vi "Process.vi"(8 "error in":errorcluster, 11 "XYStage":refnum<class "XYStage.lvclass">) -> (0 "error out":errorcluster, 3 "XYStage out":refnum<class "XYStage.lvclass">)   [LabVIEW 2020, in "XYStage.lvclass"]
doc: "---------------------------------------------------------------\nJKI State Machine Objects™\nhttp://jki.net/state-machine-objects/\nCopyright (C) 2005-2015, JKI <info@jki.net>\nALL RIGHTS RESERVEDJKI State Machine Objects (SMO) 1.0.0.5\nJKI - JKI\nCopyright (c) 2016, JKI"
uses:
  XYStage.lvclass
  XYStage.lvclass/XYStage.ctl
  <vilib>/JKI/JKI SMO/SMO/SMO.lvclass
  <vilib>/JKI/JKI SMO/SMO/Typedefs/Parent Call--Enum.ctl
  Typedefs/(real)Coords--Cluster.ctl
  C:/Program Files/National Instruments/LabVIEW 2020/vi.lib/JKI/JKI SMO/SMO/SMO.lvclass
  C:/Users/huipeng8/Desktop/SMO-HAL-Webinar/Subsystems/XYStage/XYStage.lvclass
panel:
  # "For instructions on how to use the JKI State Machine Objects, examples and video tutorials, visit:\nhttp://jki.net/state-machine-objects/\n\nJKI State Machine Objects™\nhttp://jki.net/state-machine-objects/\nCopyright (C) 2005-2015, JKI <info@jki.net>\nALL RIGHTS RESERVED"
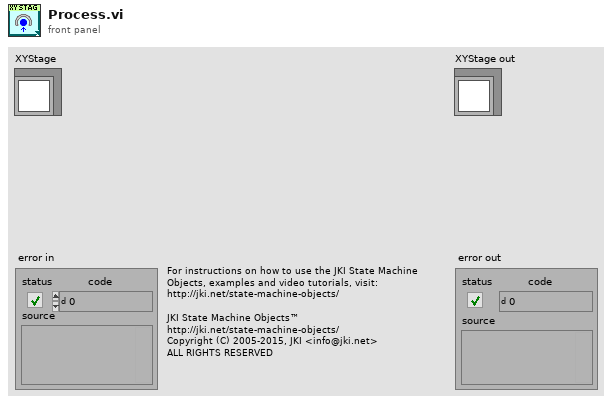
[diagram p1: front panel]
types:
  T1 = typedef "SMO.lvclass/Parent Call--Enum.ctl" = enum16{"Allows parent to run", "Does not request parent to run"}
  T2 = typedef "XYStage.lvclass/(real)Coords--Cluster.ctl" = cluster{"X":dbl, "Y":dbl}
  T3 = enum32{"invalid app kind", "Development System", "Run Time System", "Student Edition", "Embedded LabVIEW", "Evaluation", "Custom"}
  T4 = enum32{"Invalid", "Standard", "Closed", "Hidden", "Minimized", "Maximized"}
  T5 = cluster{"Core":cluster{"Current VI Reference":refnum<vi>, "Close Panel on Exit?":bool, "error":errorcluster}, "Self Reference":refnum<class "XYStage.lvclass">}
  T6 = cluster{"Current VI Reference":refnum<vi>, "Close Panel on Exit?":bool, "error":errorcluster}
  T7 = typedef "SMO.lvclass/Protected Events.ctl" = cluster{"StopProcesses":refnum<user-event>, "AbortProcesses":refnum<user-event>, "Config Changed":refnum<user-event>, "Dependency":refnum<user-event>}
  T8 = typedef "XYStage.lvclass/ProtectedEvents--Cluster.ctl" = cluster{"API_Template":refnum<user-event>}
  T9 = typedef "XYStage.lvclass/PrivateEvents--Cluster.ctl" = cluster{"MoveAbsolute":refnum<user-event>, "MoveRelative":refnum<user-event>, "MoveToNamedPosition":refnum<user-event>, "StorePosition":refnum<user-event>, "Home":refnum<user-event>}
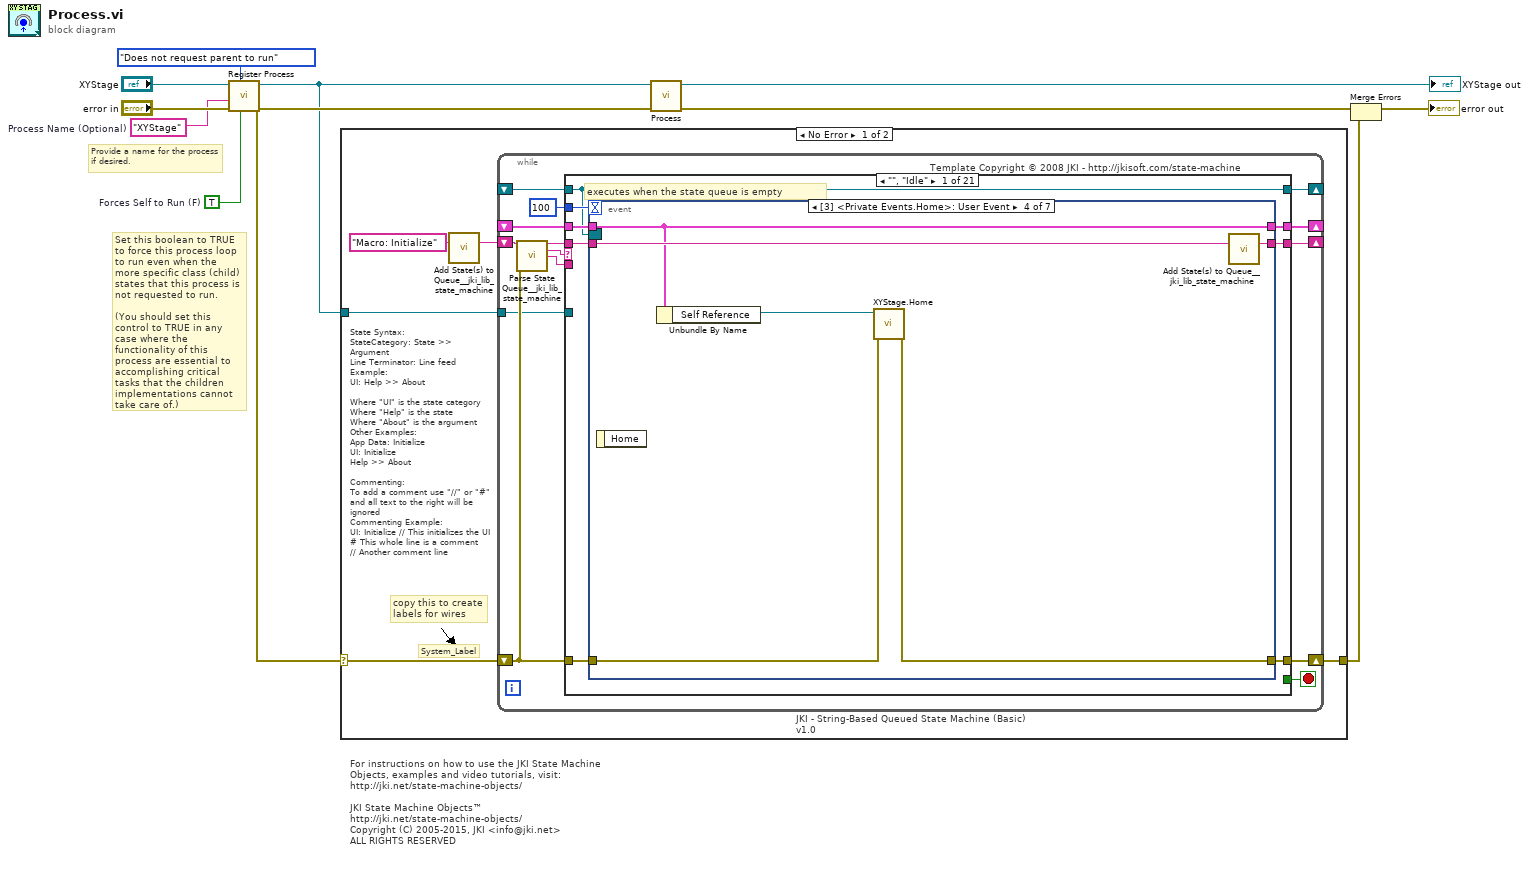
[diagram p0: block diagram]
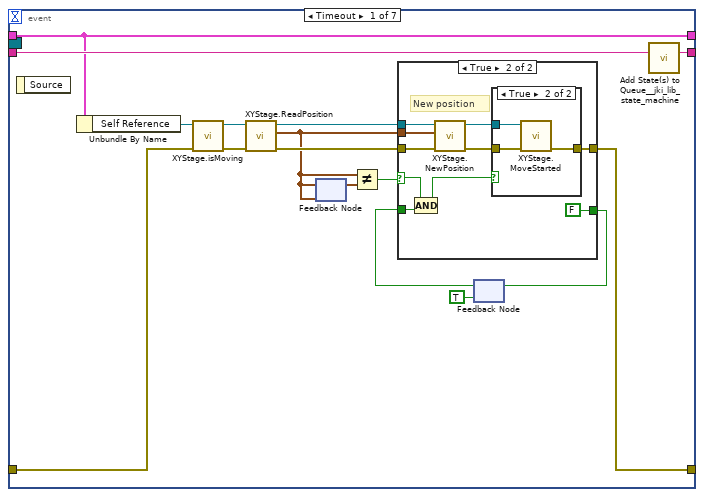
[diagram p2: hidden frame]
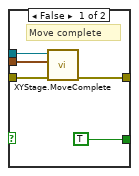
[diagram p4: hidden frame]
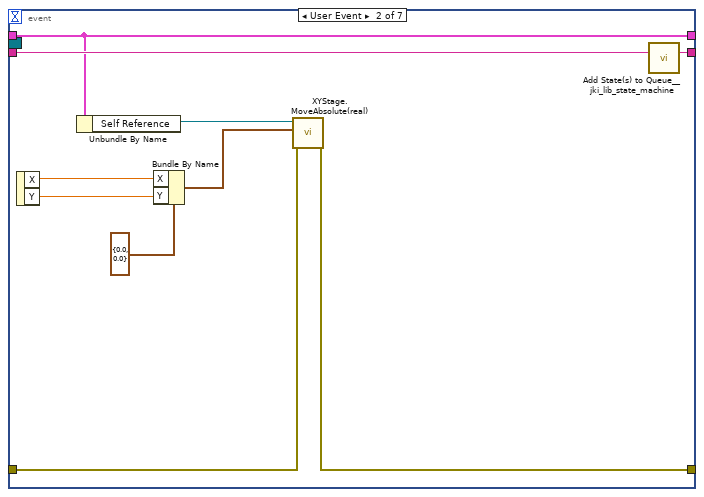
[diagram p6: hidden frame]
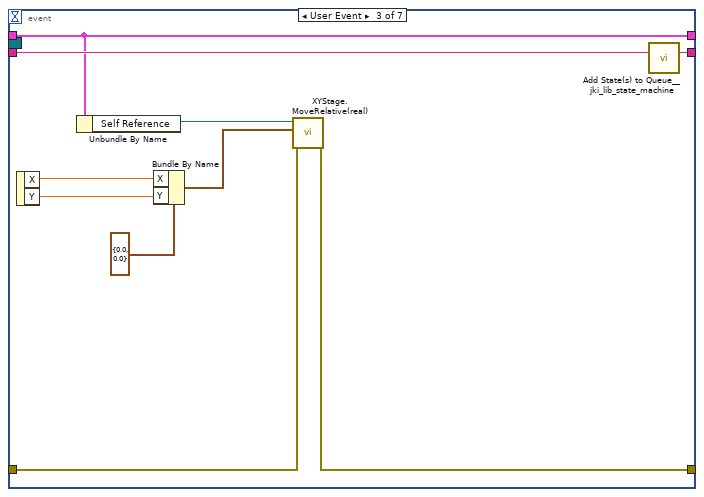
[diagram p7: hidden frame]
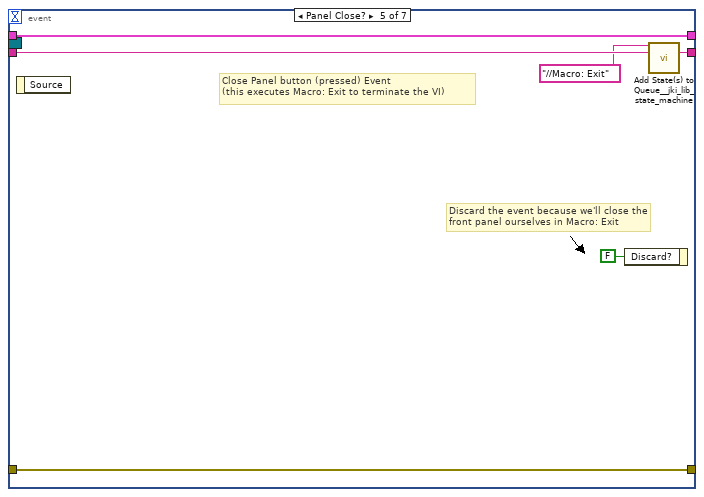
[diagram p8: hidden frame]
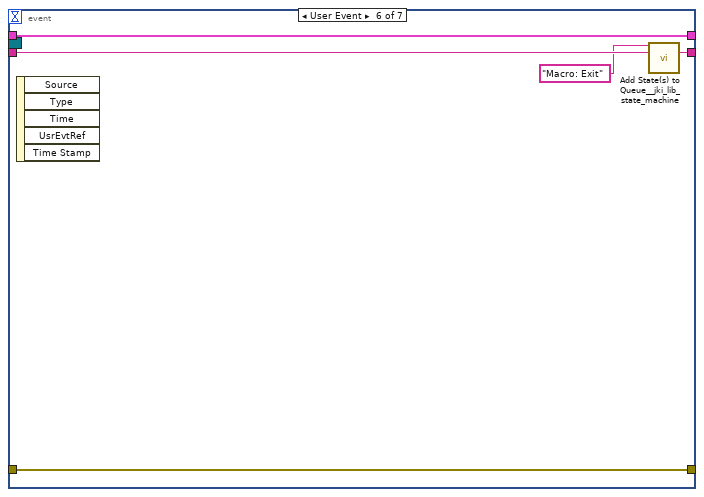
[diagram p9: hidden frame]
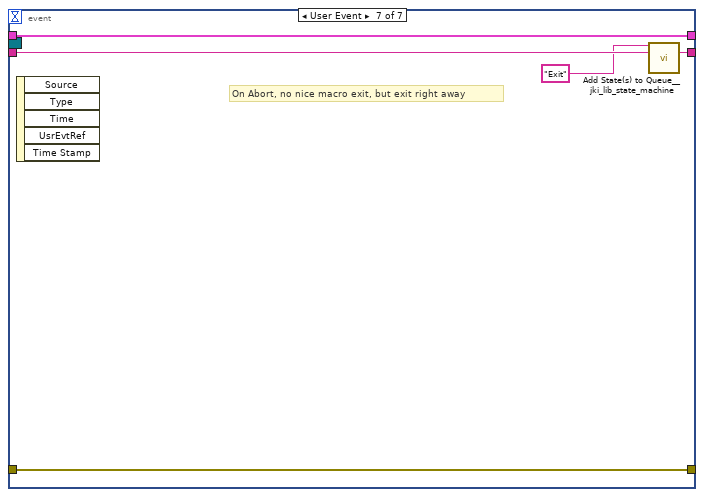
[diagram p10: hidden frame]
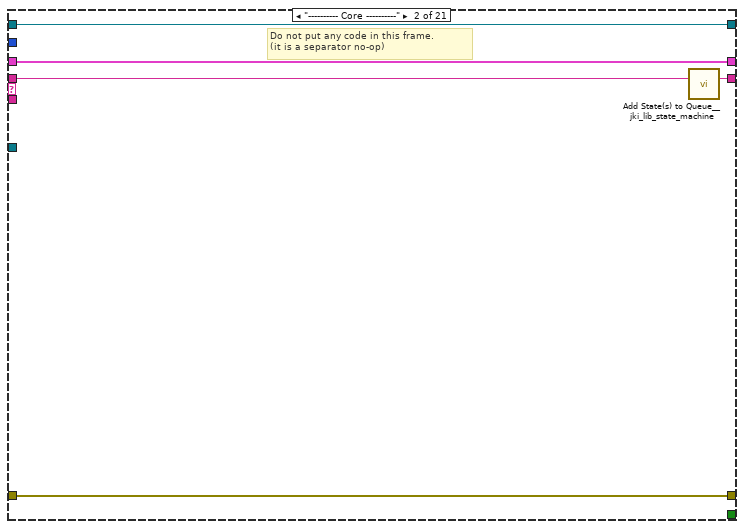
[diagram p11: hidden frame]
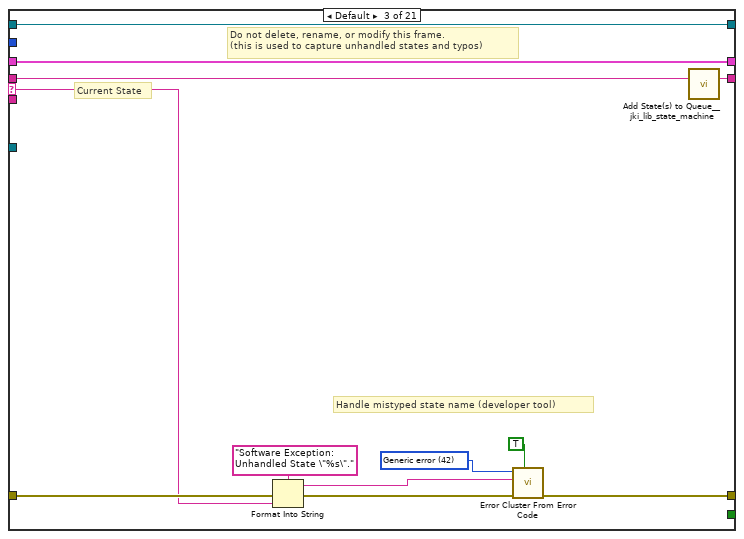
[diagram p12: hidden frame]
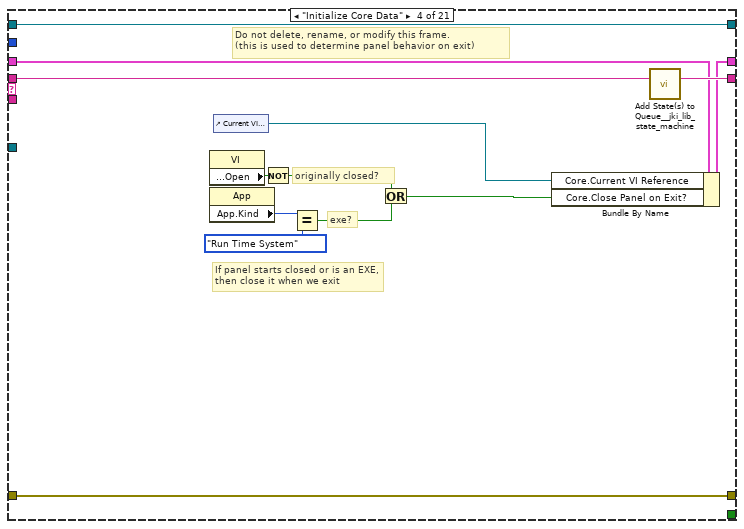
[diagram p13: hidden frame]
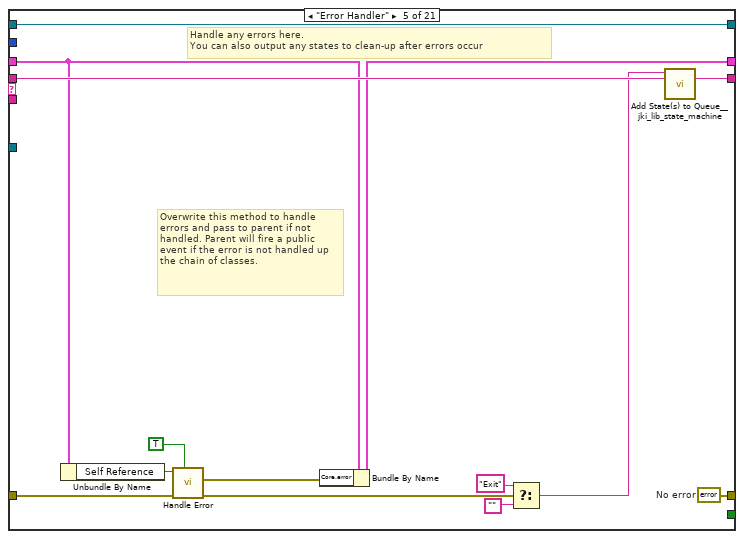
[diagram p14: hidden frame]
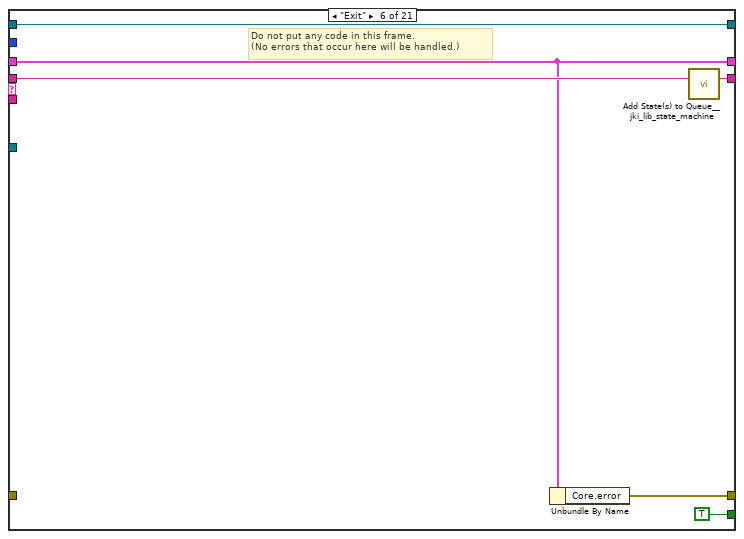
[diagram p15: hidden frame]
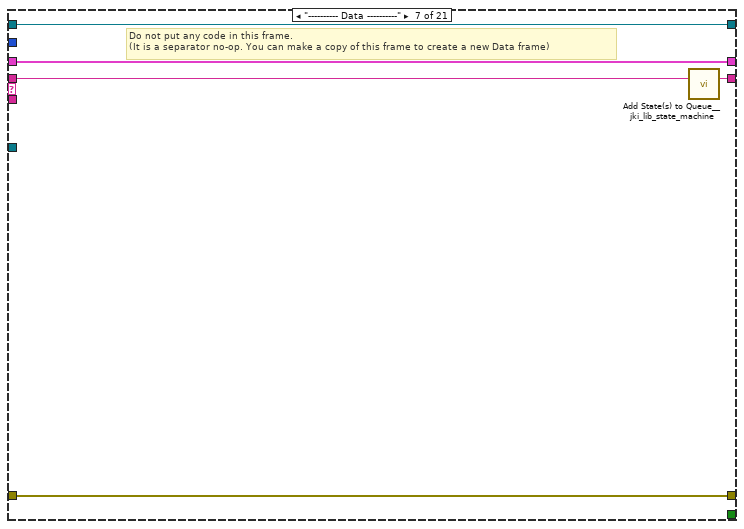
[diagram p16: hidden frame]
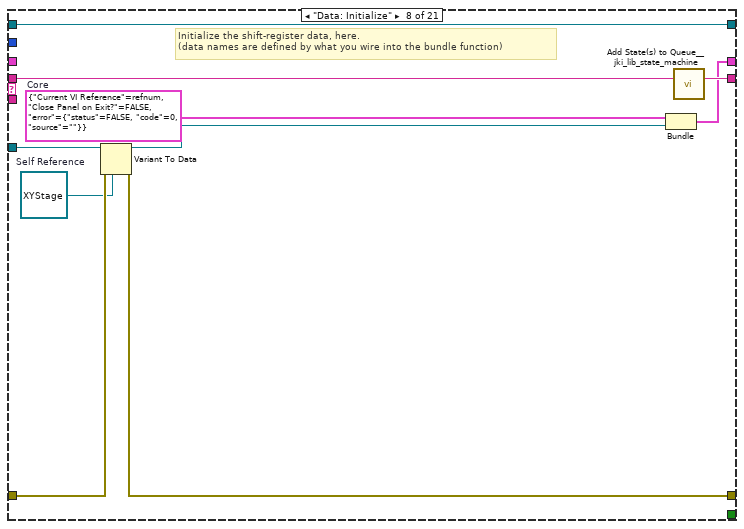
[diagram p17: hidden frame]
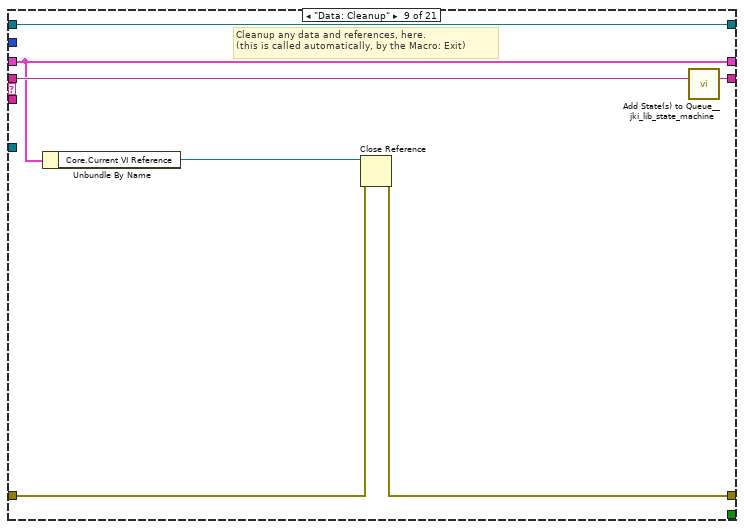
[diagram p18: hidden frame]
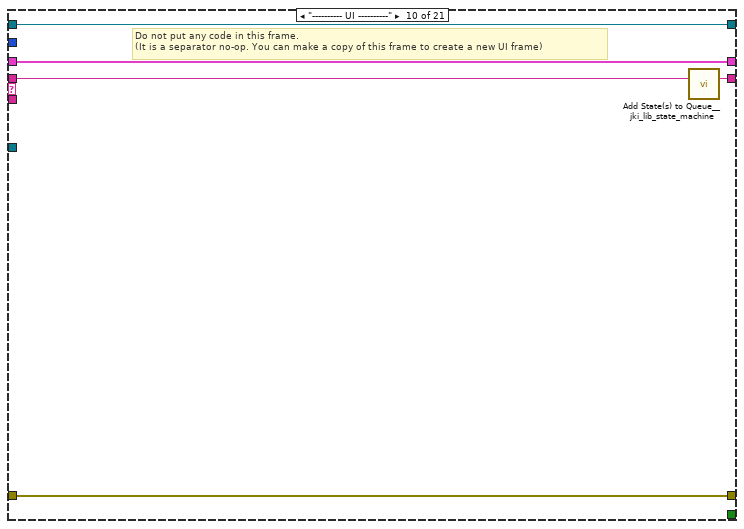
[diagram p19: hidden frame]
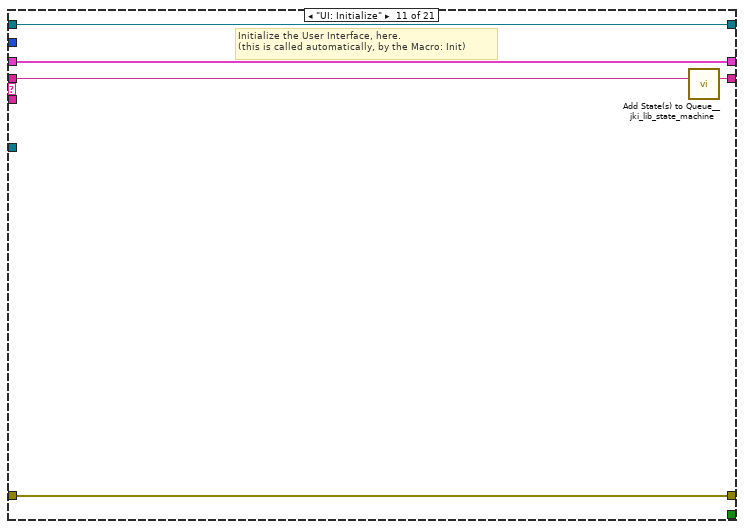
[diagram p20: hidden frame]
diagram:
  w2 = TRUE  # Forces Self to Run (F)
  w1 = "XYStage"  # Process Name (Optional)
  # "Provide a name for the process\nif desired."
  # "Set this boolean to TRUE to force this process loop to run even when the more specific class (child) states that this process is not requested to run.\n\n(You should set this control to TRUE in any case where the functionality of this process are essential to accomplishing critical tasks that the children implementations cannot take care of.)"
  # "For instructions on how to use the JKI State Machine Objects, examples and video tutorials, visit:\nhttp://jki.net/state-machine-objects/\n\nJKI State Machine Objects™\nhttp://jki.net/state-machine-objects/\nCopyright (C) 2005-2015, JKI <info@jki.net>\nALL RIGHTS RESERVED"
  n1 = call <vilib>:"Register Process.vi"("Forces Self to Run (F)"=w2, "Parent Call"=Parent_Call--Enum."Does not request parent to run", "error in (no error)"="error in", "Process Name (optional)"=w1, "SMO"="XYStage") -> ("error out"=w8:errorcluster, "SMO out"=w7:refnum<class "XYStage.lvclass">)  [unwired: 5 in]
  n2 = case shown="No Error" w8 {
    selector: w8 -> [w13 w327]
    tunnel: w7 -> [w14 _]
    tunnel: [w12 w327] -> w4
    frame No Error {
      # "State Syntax:\nStateCategory: State >> Argument\nLine Terminator: Line feed\nExample:\nUI: Help >> About\n\nWhere \"UI\" is the state category\nWhere \"Help\" is the state\nWhere \"About\" is the argument\nOther Examples:\nApp Data: Initialize\nUI: Initialize\nHelp >> About\n\nCommenting:\nTo add a comment use \"//\" or \"#\" and all text to the right will be ignored\nCommenting Example:\nUI: Initialize // This initializes the UI\n# This whole line is a comment\n// Another comment line"
      # "copy this to create labels for wires"
      # "System_Label"
      n3 = call <vilib>:"Add State(s) to Queue__jki_lib_state_machine.vi"("State(s) in (\"\")"="Macro: Initialize") -> ("States Out"=w16:string)  [unwired: 14 in]
      n4 = while "JKI - String-Based Queued State Machine (Basic) v1.0" {
        shift-right: [w23] -> _
        shift-left: _ -> [w22]
        shift-right: [w26] -> w12
        shift-left: w13 -> [w20]
        shift-right: [w25] -> _
        shift-left: w16 -> [w27]
        tunnel: w14 -> [w19]
        shift-right: [w18] -> _
        shift-left: _ -> [w17]
        stop <- w24 stop-if-true
        # "Template Copyright © 2008 JKI - http://jkisoft.com/state-machine"
        n5 = call <vilib>:"Parse State Queue__jki_lib_state_machine.vi"("State Queue"=w27, "Error In (no error)"=w20) -> ("Remaining States"=w29:string, "Current State"=w30:string, "Arguments"=w28:string)  [unwired: 11 in]
        n6 = case shown="\"\", \"Idle\"" w30 {
          selector: w30 -> [_ _ w130 _ _ _ _ _ _ _ _ _ _ _ _ _ _ _ _ _ _]
          tunnel: w29 -> [w38 w128 w134 w153 w167 w173 w178 w188 w195 w200 w205 w212 w228 w260 w269 w283 w288 w299 w304 w320 w326]
          tunnel: w28 -> [_ _ _ _ _ _ _ _ _ _ _ w206 w222 _ _ _ _ _ _ _ _]
          tunnel: w22 -> [w36 w125 w132 w144 w156 w169 w175 _ w190 w197 w203 w210 w224 w257 w265 w274 w285 w296 w301 w318 w324]
          tunnel: [w35 w126 w136 w150 w158 w168 w176 w184 w191 w198 w202 w207 w225 w258 w267 w281 w286 w290 w302 w307 w322] -> w26
          tunnel: w20 -> [w34 w126 w135 w150 w163 _ w176 w185 w192 w198 w202 w208 w226 w258 w267 w281 w286 w291 w302 w310 w322]
          tunnel: [w37 w127 w133 w152 w166 w172 w177 w187 w194 w199 w204 w211 w227 w259 w268 w282 w287 w298 w303 w319 w325] -> w25
          tunnel: [_ _ _ _ _ TRUE _ _ _ _ _ _ _ _ _ _ _ _ _ _ _] -> w24
          tunnel: [w33 w125 w132 w151 w155 w169 w175 w186 w190 w197 w203 w210 w224 w257 w265 w274 w285 w296 w301 w318 w324] -> w23
          tunnel: 100 ("Timeout") -> [w32 _ _ _ _ _ _ _ _ _ _ _ _ _ _ _ _ _ _ _ _]
          tunnel: w19 -> [_ _ _ _ _ _ _ w182 _ _ _ _ _ _ _ _ _ _ _ _ _]
          tunnel: [w31 w124 w129 w141 w165 w170 w174 w180 w189 w196 w201 w209 w221 w256 w266 w275 w284 w297 w300 w317 w323] -> w18
          tunnel: w17 -> [w31 w124 w129 w141 w165 w170 w174 w180 w189 w196 w201 w209 w221 w256 w266 w275 w284 w297 w300 _ w323]
          frame "", "Idle" {
            # "executes when the state queue is empty"
            n7 = event shown="[3] <Private Events.Home>: User Event" {
              selector: w31 -> [_ _ _ _ _ _ _]
              dyn-events: _ -> [_ _ _ _ _ _ _]
              timeout: w32 -> [_ _ _ _ _ _ _]
              tunnel: w38 -> [w54 w91 w101 w107 w113 w118 w123]
              tunnel: [w53 w90 w100 w106 w112 w117 w122] -> w37
              tunnel: w36 -> [w52 w89 w99 w105 w110 w115 w120]
              tunnel: [w46 w82 w92 w102 w111 w116 w121] -> w35
              tunnel: w34 -> [w43 w83 w93 w103 w111 w116 w121]
              tunnel: [w52 w89 w99 w105 w110 w115 w120] -> w33
              event Timeout {
                n8 = event-data() -> ()  [unwired: 1 in, 1 out]
                n9 = Unbundle By Name(w52) -> ("Self Reference"=w45:refnum<class "XYStage.lvclass">)
                n10 = call-dynamic "XYStage.isMoving.vi"("error in (no error)"=w43, "XYStage"=w45) -> ("error out"=w42:errorcluster, "XYStage out"=w44:refnum<class "XYStage.lvclass">)  [unwired: 7 in, 1 out]
                n11 = call-dynamic "XYStage.ReadPosition.vi"("error in (no error)"=w42, "XYStage"=w44) -> ("error out"=w50:errorcluster, "Position"=w48:T2, "XYStage out"=w51:refnum<class "XYStage.lvclass">)  [unwired: 6 in, 1 out]
                n12 = feedback-in #1(w48) -> ()
                n13 = feedback #1(w48) -> (w49:T2)
                n14 = Not Equal?(x=w48, y=w49) -> (x != y?=w47:bool)
                n15 = feedback #2(TRUE) -> (w39:bool)
                n16 = case shown="True" w47 {
                  selector: w47 -> [_ w72]
                  tunnel: w51 -> [w60 w77]
                  tunnel: w50 -> [w58 w76]
                  tunnel: w48 -> [w59 w75]
                  tunnel: [w57 w68] -> w46
                  tunnel: [w56 FALSE] -> w41
                  tunnel: w39 -> [w55 w73]
                  frame False {
                    n17 = case shown="True" w55 {
                      selector: w55 -> [_ w67]
                      tunnel: w60 -> [w65 _]
                      tunnel: w59 -> [w64 _]
                      tunnel: w58 -> [w63 w66]
                      tunnel: [w62 w66] -> w57
                      tunnel: [TRUE w67] -> w56
                      frame False {
                        # "Move complete"
                        n18 = call "XYStage.MoveComplete.vi"("error in (no error)"=w63, "Coords"=w64, "XYStage"=w65) -> ("error out"=w62:errorcluster)  [unwired: 7 in, 1 out]
                      }
                      frame True {
                      }
                    }
                  }
                  frame True {
                    # "New position"
                    n19 = Compound Arithmetic op=AND(w72, w73) -> (w71:bool)
                    n20 = call "XYStage.NewPosition.vi"("error in (no error)"=w76, "Position"=w75, "XYStage"=w77) -> ("error out"=w69:errorcluster, "XYStage out"=w70:refnum<class "XYStage.lvclass">)  [unwired: 7 in]
                    n21 = case shown="True" w71 {
                      tunnel: w70 -> [_ w81]
                      tunnel: w69 -> [w78 w80]
                      tunnel: [w78 w79] -> w68
                      frame False {
                      }
                      frame True {
                        n22 = call "XYStage.MoveStarted.vi"("error in (no error)"=w80, "XYStage"=w81) -> ("error out"=w79:errorcluster)  [unwired: 8 in, 1 out]
                      }
                    }
                  }
                }
                n23 = feedback-in #2(w41) -> ()
                n24 = call <vilib>:"Add State(s) to Queue__jki_lib_state_machine.vi"("State(s) in (\"\")"=w54) -> ("States Out"=w53:string)  [unwired: 14 in]
              }
              event User Event {
                n25 = event-data() -> ("X"=w86:dbl, "Y"=w87:dbl)  [unwired: 1 in]
                n26 = Unbundle By Name(w89) -> ("Self Reference"=w84:refnum<class "XYStage.lvclass">)
                n27 = Bundle By Name(cluster=T2 {"X"=0.0, "Y"=0.0} ("Coords"), "X"=w86, "Y"=w87) -> (w85:T2)
                n28 = call-dynamic "XYStage.MoveAbsolute(real).vi"("error in (no error)"=w83, "Position"=w85, "XYStage"=w84) -> ("error out"=w82:errorcluster)  [unwired: 6 in, 2 out]
                n29 = call <vilib>:"Add State(s) to Queue__jki_lib_state_machine.vi"("State(s) in (\"\")"=w91) -> ("States Out"=w90:string)  [unwired: 14 in]
              }
              event User Event {
                n30 = event-data() -> ("X"=w96:dbl, "Y"=w97:dbl)  [unwired: 1 in]
                n31 = Unbundle By Name(w99) -> ("Self Reference"=w95:refnum<class "XYStage.lvclass">)
                n32 = Bundle By Name(cluster=T2 {"X"=0.0, "Y"=0.0} ("Coords"), "X"=w96, "Y"=w97) -> (w94:T2)
                n33 = call-dynamic "XYStage.MoveRelative(real).vi"("error in (no error)"=w93, "Relative Units"=w94, "XYStage"=w95) -> ("error out"=w92:errorcluster)  [unwired: 6 in, 2 out]
                n34 = call <vilib>:"Add State(s) to Queue__jki_lib_state_machine.vi"("State(s) in (\"\")"=w101) -> ("States Out"=w100:string)  [unwired: 14 in]
              }
              event User Event {
                n35 = event-data() -> ()  [unwired: 1 in, 1 out]
                n36 = Unbundle By Name(w105) -> ("Self Reference"=w104:refnum<class "XYStage.lvclass">)
                n37 = call-dynamic "XYStage.Home.vi"("error in (no error)"=w103, "XYStage"=w104) -> ("error out"=w102:errorcluster)  [unwired: 8 in, 1 out]
                n38 = call <vilib>:"Add State(s) to Queue__jki_lib_state_machine.vi"("State(s) in (\"\")"=w107) -> ("States Out"=w106:string)  [unwired: 14 in]
              }
              event Panel Close? {
                # "Discard the event because we'll close the front panel ourselves in Macro: Exit"
                # "Close Panel button (pressed) Event\n(this executes Macro: Exit to terminate the VI)"
                n39 = event-data() -> ()  [unwired: 1 in, 1 out]
                n40 = event-data("Discard?"=FALSE) -> ()  [unwired: 1 in, 1 out]
                n41 = call <vilib>:"Add State(s) to Queue__jki_lib_state_machine.vi"("State(s) in Front (\"\")"="//Macro: Exit", "State(s) in (\"\")"=w113) -> ("States Out"=w112:string)  [unwired: 13 in]
              }
              event User Event {
                n42 = event-data() -> ()  [unwired: 1 in, 5 out]
                n43 = call <vilib>:"Add State(s) to Queue__jki_lib_state_machine.vi"("State(s) in Front (\"\")"="Macro: Exit", "State(s) in (\"\")"=w118) -> ("States Out"=w117:string)  [unwired: 13 in]
              }
              event User Event {
                # "On Abort, no nice macro exit, but exit right away"
                n44 = event-data() -> ()  [unwired: 1 in, 5 out]
                n45 = call <vilib>:"Add State(s) to Queue__jki_lib_state_machine.vi"("State(s) in Front (\"\")"="Exit", "State(s) in (\"\")"=w123) -> ("States Out"=w122:string)  [unwired: 13 in]
              }
            }
          }
          frame "---------- Core ----------" {
            # "Do not put any code in this frame.\n(it is a separator no-op)"
            n46 = call <vilib>:"Add State(s) to Queue__jki_lib_state_machine.vi"("State(s) in (\"\")"=w128) -> ("States Out"=w127:string)  [unwired: 14 in]
          }
          frame Default {
            w139 = 42 items=["No error", "Argument error", "Memory is full", "Out of zone", "End of file", "File already open", "Generic file I/O error", "File not found", "File permission error", "Disk is full", "Duplicate path", "Too many files open", "System feature not enabled", "Resource file not found", "Cannot add resource", "Resource not found", "Image not found", "Image memory error", "Pen does not exist", "Config type invalid", "Config token not found", "Config parse error", "Config memory error", "Bad external code format", "Bad external code offset", "External code not present", "Null window", "Destroy window error", "Null menu", "Print aborted", "Bad print record", "Print driver error", "Windows error during printing", "Memory error during printing", "Print dialog error", "Generic print error", "Invalid device refnum", "Device not found", "Device parameter error", "Device unit error", "Cannot open device", "Device call aborted", "Generic error", "Cancelled by user", "Object ID too low", "Object ID too high", "Object not in heap", "Unknown heap", "Unknown object (invalid DefProc)", "Unknown object (DefProc not in table)", "Message out of range", "Invalid (null) method", "Unknown message", "Manager call not supported", "Bad address", "Network operation in progress", "Network operation timed out", "Connection is busy", "Network attribute not supported", "Network error", "Address in use", "System out of memory", "Connection aborted", "Connection refused", "Not connected", "Already connected", "Connection closed", "Initialization error (interapplication manager)", "Bad occurrence", "Wait on unbound occurrence handler", "Occurrence queue overflow", "Datalog type conflict", "Unused", "Unrecognized type (interapplication manager)", "Memory corrupt", "Failed to make temporary DLL", "Old CIN version", "Drag socket not found", "Failed to load drop-object", "Failed to register OLE object", "Failed to release OLE object", "Format specifier type mismatch", "Unknown format specifier", "Too few format specifiers", "Too many format specifiers", "Scan failed", "Newer CIN version", "Error converting to variant", "Runtime menu error", "Password tampered", "Variant attribute not found", "Incompatible variant data type", "Event data is not available", "Event Store is not present", "Occurrence is not found", "Event Queue is not created", "Event info is not available", "Refnum passed is NULL", "Error retrieving Class GUID", "Error retrieving CoClass GUID", "Error retrieving TypeLib GUID.", "Bad built application magic bytes.", "Specific driver is different from the specific driver associated with the Logical Name.", "There is no session opened to the class driver.", "Max Error", "MAX - Error with config objects", "MAX - Error loading configuration", "MAX - Group not supported"]
            # "Current State"
            # "Do not delete, rename, or modify this frame.\n(this is used to capture unhandled states and typos)"
            # "Handle mistyped state name (developer tool)"
            n47 = Format Into String(format string="Software Exception: Unhandled State \"%s\"." ("message"), error in=w135, w130) -> (resulting string=w138:string, error out=w137:errorcluster)  [unwired: 1 in]
            n48 = call <vilib>:"Error Cluster From Error Code.vi"("show call chain? (False)"=TRUE, "error in (no error)"=w137, "error message (\"\")"=w138, "error code (0)"=w139) -> ("error out"=w136:errorcluster)  [unwired: 5 in]
            n49 = call <vilib>:"Add State(s) to Queue__jki_lib_state_machine.vi"("State(s) in (\"\")"=w134) -> ("States Out"=w133:string)  [unwired: 14 in]
          }
          frame "Initialize Core Data" {
            # "Do not delete, rename, or modify this frame.\n(this is used to determine panel behavior on exit)"
            # "originally closed?"
            # "exe?"
            # "If panel starts closed or is an EXE, then close it when we exit"
            n50 = property class="VI"() -> ("Front Panel.Open"=w149:bool)  [unwired: 2 in, 2 out]
            n51 = property class="App"() -> ("App.Kind"=w148:T3)  [unwired: 2 in, 2 out]
            n52 = control-ref of="Current VI Reference"() -> (w142:refnum<vi>)
            n53 = Not(x=w149) -> (.not. x?=w146:bool)
            n54 = Equal?(x=w148, y=T3."Run Time System" ("Application:Kind")) -> (x = y?=w145:bool)
            n55 = Or(x=w146, y=w145) -> (x .or. y?=w143:bool)
            n56 = Bundle By Name(cluster=w144, "Core.Current VI Reference"=w142, "Core.Close Panel on Exit?"=w143) -> (w151:T5)
            n57 = call <vilib>:"Add State(s) to Queue__jki_lib_state_machine.vi"("State(s) in (\"\")"=w153) -> ("States Out"=w152:string)  [unwired: 14 in]
          }
          frame "Error Handler" {
            w158 = errorcluster {"status"=FALSE, "code"=0, "source"=""}  # No error
            # "Overwrite this method to handle errors and pass to parent if not handled. Parent will fire a public event if the error is not handled up the chain of classes."
            # "Handle any errors here.\nYou can also output any states to clean-up after errors occur"
            n58 = Unbundle By Name(w156) -> ("Self Reference"=w164:refnum<class "XYStage.lvclass">)
            n59 = call-dynamic "Handle Error.vi"("Stop on Unhandled Error (T)"=TRUE, "error in"=w163, "SMO"=w164) -> ("handling error"=w159:errorcluster, "Unhandled error"=w157:errorcluster)  [unwired: 6 in, 1 out]
            n60 = Bundle By Name(cluster=w156, "Core.error"=w157) -> (w155:T5)
            n61 = Select(t="Exit", s=w159, f="") -> (s? t:f=w160:string)
            n62 = call <vilib>:"Add State(s) to Queue__jki_lib_state_machine.vi"("State(s) in Front (\"\")"=w160, "State(s) in (\"\")"=w167) -> ("States Out"=w166:string)  [unwired: 13 in]
          }
          frame "Exit" {
            # "Do not put any code in this frame.\n(No errors that occur here will be handled.)"
            n63 = Unbundle By Name(w169) -> ("Core.error"=w168:errorcluster)
            n64 = call <vilib>:"Add State(s) to Queue__jki_lib_state_machine.vi"("State(s) in (\"\")"=w173) -> ("States Out"=w172:string)  [unwired: 14 in]
          }
          frame "---------- Data ----------" {
            # "Do not put any code in this frame.\n(It is a separator no-op. You can make a copy of this frame to create a new Data frame)"
            n65 = call <vilib>:"Add State(s) to Queue__jki_lib_state_machine.vi"("State(s) in (\"\")"=w178) -> ("States Out"=w177:string)  [unwired: 14 in]
          }
          frame "Data: Initialize" {
            w179 = T6 {"Current VI Reference"=refnum, "Close Panel on Exit?"=FALSE, "error"={"status"=FALSE, "code"=0, "source"=""}}  # Core
            w183 = refnum<class "XYStage.lvclass"> refnum  # Self Reference
            # "Initialize the shift-register data, here.\n(data names are defined by what you wire into the bundle function)"
            n66 = Variant To Data(error in=w185, type=w183, Variant=w182) -> (data=w181:refnum<class "XYStage.lvclass">, error out=w184:errorcluster)
            n67 = Bundle("Core"=w179, "Self Reference"=w181) -> (w186:T5)  [unwired: 1 in]
            n68 = call <vilib>:"Add State(s) to Queue__jki_lib_state_machine.vi"("State(s) in (\"\")"=w188) -> ("States Out"=w187:string)  [unwired: 14 in]
          }
          frame "Data: Cleanup" {
            # "Cleanup any data and references, here.\n(this is called automatically, by the Macro: Exit)"
            n69 = Unbundle By Name(w190) -> ("Core.Current VI Reference"=w193:refnum<vi>)
            n70 = Close Reference(reference=w193, error in (no error)=w192) -> (error out=w191:errorcluster)
            n71 = call <vilib>:"Add State(s) to Queue__jki_lib_state_machine.vi"("State(s) in (\"\")"=w195) -> ("States Out"=w194:string)  [unwired: 14 in]
          }
          frame "---------- UI ----------" {
            # "Do not put any code in this frame.\n(It is a separator no-op. You can make a copy of this frame to create a new UI frame)"
            n72 = call <vilib>:"Add State(s) to Queue__jki_lib_state_machine.vi"("State(s) in (\"\")"=w200) -> ("States Out"=w199:string)  [unwired: 14 in]
          }
          frame "UI: Initialize" {
            # "Initialize the User Interface, here.\n(this is called automatically, by the Macro: Init)"
            n73 = call <vilib>:"Add State(s) to Queue__jki_lib_state_machine.vi"("State(s) in (\"\")"=w205) -> ("States Out"=w204:string)  [unwired: 14 in]
          }
          frame "UI: Cursor Set" {
            # "Argument"
            # "Initialize the User Interface, here.\n(this is called automatically, by the Macro: Init)"
            n74 = disable-structure shown="Default" {
              disable-tunnel: w208 -> [w213 w216]
              disable-tunnel: [w213 w215] -> w207
              disable-tunnel: w206 -> [_ w214]
              frame condition #0 {
              }
              frame condition #1 (active) {
                n75 = case shown="\"Idle\", Default" w214 {
                  tunnel: w216 -> [w218 w220]
                  tunnel: [w217 w219] -> w215
                  frame "Idle", Default {
                    n76 = call <vilib>:"Unset Busy.vi"("error in (no error)"=w218) -> ("error out"=w217:errorcluster)  [unwired: 10 in]
                  }
                  frame "Busy" {
                    n77 = call <vilib>:"Set Busy.vi"("error in (no error)"=w220) -> ("error out"=w219:errorcluster)  [unwired: 9 in, 1 out]
                  }
                }
              }
            }
            n78 = call <vilib>:"Add State(s) to Queue__jki_lib_state_machine.vi"("State(s) in (\"\")"=w212) -> ("States Out"=w211:string)  [unwired: 14 in]
          }
          frame "UI: Front Panel State" {
            # "Argument"
            # "Set Front Panel Open or Closed\n(Usage: \"UI: Front Panel State >> Open|Close\")"
            n79 = Unbundle By Name(w224) -> ("Core.Current VI Reference"=w223:refnum<vi>)
            n80 = disable-structure shown="Default" {
              disable-tunnel: w226 -> [w232 w255]
              disable-tunnel: [w231 w255] -> w225
              disable-tunnel: w223 -> [w230 _]
              disable-tunnel: w222 -> [w229 _]
              frame condition #0 (active) {
                n81 = case shown="\"Close\"" w229 {
                  tunnel: w232 -> [w236 w249]
                  tunnel: [w238 w250] -> w231
                  tunnel: w230 -> [w237 w247]
                  frame "Open", Default {
                    n82 = property class="VI"(reference=w237, error in=w236) -> (reference out=w234:refnum<vi>, error out=w235:errorcluster, "FP.State"=w233:T4)
                    n83 = case shown="\"Closed\"" w233 {
                      tunnel: [w241 w244] -> w238
                      tunnel: w235 -> [w240 w244]
                      tunnel: w234 -> [w239 _]
                      frame "Closed" {
                        n84 = invoke class="VI" method="FP.Open"(reference=w239, error in=w240, "Activate"=TRUE, "State"=T4."Standard") -> (error out=w241:errorcluster)  [unwired: 1 in, 4 out]
                      }
                      frame Default {
                      }
                    }
                  }
                  frame "Close" {
                    n85 = property class="VI"(reference=w247, error in=w249) -> (reference out=w246:refnum<vi>, error out=w248:errorcluster, "FP.State"=w245:T4)
                    n86 = case shown="Default" w245 {
                      tunnel: [w251 w254] -> w250
                      tunnel: w248 -> [w251 w253]
                      tunnel: w246 -> [_ w252]
                      frame "Invalid", "Closed" {
                      }
                      frame Default {
                        n87 = invoke class="VI" method="FP.Close"(reference=w252, error in=w253) -> (error out=w254:errorcluster)  [unwired: 1 in, 2 out]
                      }
                    }
                  }
                }
              }
              frame condition #1 {
              }
            }
            n88 = call <vilib>:"Add State(s) to Queue__jki_lib_state_machine.vi"("State(s) in (\"\")"=w228) -> ("States Out"=w227:string)  [unwired: 14 in]
          }
          frame "---------- Macro ----------" {
            # "Do not put any code in this frame.\n(It is a separator no-op. You can make a copy of this frame to create a new Macro frame)"
            n89 = call <vilib>:"Add State(s) to Queue__jki_lib_state_machine.vi"("State(s) in (\"\")"=w260) -> ("States Out"=w259:string)  [unwired: 14 in]
          }
          frame "Macro: Initialize" {
            w263 = "UI: Initialize\n//UI: Front Panel State >> Open"  # UI: Initialize //UI: Front Panel State >> Open
            # "Initialization Macro\n(This is called once, when the VI starts)"
            n90 = call <vilib>:"Add State(s) to Queue__jki_lib_state_machine.vi"("State(s) in Front (\"\")"="Data: Initialize\nInitialize Core Data\nEvents: Register", "State(s) in (\"\")"="Process: Sync", "State(s) at Back (\"\")"=w263) -> ("States Out"=w262:string)  [unwired: 12 in]
            n91 = call <vilib>:"Add State(s) to Queue__jki_lib_state_machine.vi"("State(s) in Front (\"\")"=w262, "State(s) in (\"\")"=w269) -> ("States Out"=w268:string)  [unwired: 13 in]
          }
          frame "Macro: Exit" {
            # "Exit Macro\n(This is called once, when the VI exits)"
            n92 = Unbundle By Name(w274) -> ("Core.Close Panel on Exit?"=w280:bool)
            n93 = Select(t="UI: Front Panel State >> Close", s=w280, f="") -> (s? t:f=w277:string)
            n94 = call <vilib>:"Add State(s) to Queue__jki_lib_state_machine.vi"("State(s) in Front (\"\")"="Data: Cleanup\nEvents: Unregister", "State(s) in (\"\")"="Process: Sync", "State(s) at Back (\"\")"="Exit") -> ("States Out"=w271:string)  [unwired: 12 in]
            n95 = call <vilib>:"Add State(s) to Queue__jki_lib_state_machine.vi"("State(s) in (\"\")"=w277, "State(s) at Back (\"\")"=w271) -> ("States Out"=w276:string)  [unwired: 13 in]
            n96 = call <vilib>:"Add State(s) to Queue__jki_lib_state_machine.vi"("State(s) in Front (\"\")"=w276, "State(s) in (\"\")"=w283) -> ("States Out"=w282:string)  [unwired: 13 in]
          }
          frame "---------- Process ----------" {
            # "Template Separator\n(You can make a copy of, or modify, this frame)"
            n97 = call <vilib>:"Add State(s) to Queue__jki_lib_state_machine.vi"("State(s) in (\"\")"=w288) -> ("States Out"=w287:string)  [unwired: 14 in]
          }
          frame "Process: Sync" {
            n98 = Unbundle By Name(w296) -> ("Self Reference"=w292:refnum<class "XYStage.lvclass">)
            n99 = call <vilib>:"WaitOnProcessSync.vi"("error in (no error)"=w291, "SMO"=w292) -> ("error out"=w290:errorcluster, "Don't run?"=w295:bool)  [unwired: 7 in, 1 out]
            n100 = Select(t="Data: Cleanup\nEvents: Unregister\nExit", s=w295, f="") -> (s? t:f=w289:string)
            n101 = call <vilib>:"Add State(s) to Queue__jki_lib_state_machine.vi"("State(s) in Front (\"\")"=w289, "State(s) in (\"\")"=w299) -> ("States Out"=w298:string)  [unwired: 13 in]
          }
          frame "---------- Events ----------" {
            # "Template Separator\n(You can make a copy of, or modify, this frame)"
            n102 = call <vilib>:"Add State(s) to Queue__jki_lib_state_machine.vi"("State(s) in (\"\")"=w304) -> ("States Out"=w303:string)  [unwired: 14 in]
          }
          frame "Events: Register" {
            # "Expand to add\nmore events"
            # "Self Events (API Calls)"
            # "Base Class Protected Events"
            n103 = Unbundle By Name(w318) -> ("Self Reference"=w313:refnum<class "XYStage.lvclass">)
            n104 = call <vilib>:"GetProtectedEvents.vi"("SMO"=w313) -> ("error out"=w305:errorcluster, "SMO Protected Events"=w316:T7, "SMO out"=w315:refnum<class "XYStage.lvclass">)  [unwired: 8 in]
            n105 = call "XYStage.GetProtectedEvents.vi"("XYStage"=w315) -> ("error out"=w306:errorcluster, "Protected Events"=w314:T8, "XYStage out"=w312:refnum<class "XYStage.lvclass">)  [unwired: 8 in]
            n106 = call "XYStage.GetPrivateEvents.vi"("XYStage"=w312) -> ("error out"=w309:errorcluster, "Private Events"=w311:T9)  [unwired: 8 in, 1 out]
            n107 = register-events(w316, w314, w311) -> (reference out=w317:refnum<event-registration>, error out=w308:errorcluster)  [unwired: 2 in]
            n108 = Merge Errors(w310, w308, w309, w306, w305) -> (w307:errorcluster)
            n109 = call <vilib>:"Add State(s) to Queue__jki_lib_state_machine.vi"("State(s) in (\"\")"=w320) -> ("States Out"=w319:string)  [unwired: 14 in]
          }
          frame "Events: Unregister" {
            n110 = Unregister For Events(event registration refnum=w323, error in=w322) -> (error out=w321:errorcluster)
            n111 = call <vilib>:"Clear Errors.vi"("error in (no error)"=w321) -> ()  [unwired: 5 in, 2 out]
            n112 = call <vilib>:"Add State(s) to Queue__jki_lib_state_machine.vi"("State(s) in (\"\")"=w326) -> ("States Out"=w325:string)  [unwired: 14 in]
          }
        }
      }
    }
    frame Error {
    }
  }
  n113 = call-parent "Process.vi"("error in"=w8, "SMO"=w7) -> ("error out"=w5:errorcluster, "SMO out"=→"XYStage out":refnum<class "XYStage.lvclass">)  [unwired: 8 in]
  n114 = Merge Errors(w5, w4) -> (→"error out":errorcluster)
